vi "Place dots.vi"(6 "Right width (IMAQ height)":dbl, 8 "Left width (IMAQ height)":dbl, 9 "Right Corner":cluster{"X":sgl, "Y":sgl}[](array[cluster]), 10 "Left Corner":cluster{"X":sgl, "Y":sgl}[](array[cluster]), 11 "Image IN":T1) -> (3 "Image OUT":T1)   [LabVIEW 2018]
uses:
  <vilib>/vision/Image Controls.llb/IMAQ Image.ctl
  Dashboard globals.vi
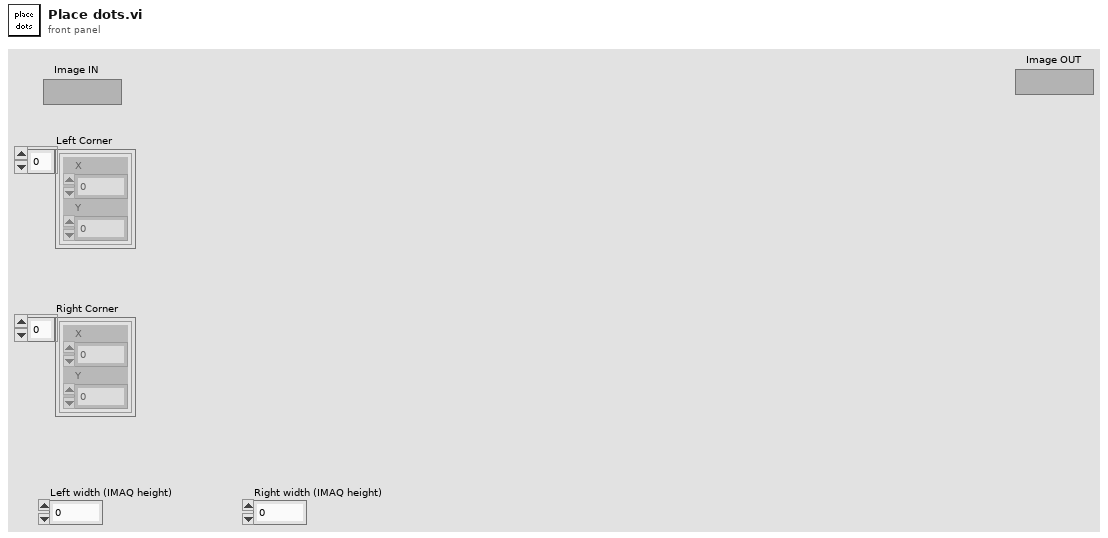
[diagram p1: front panel]
types:
  T1 = typedef "IMAQ Image.ctl" = refnum<image>
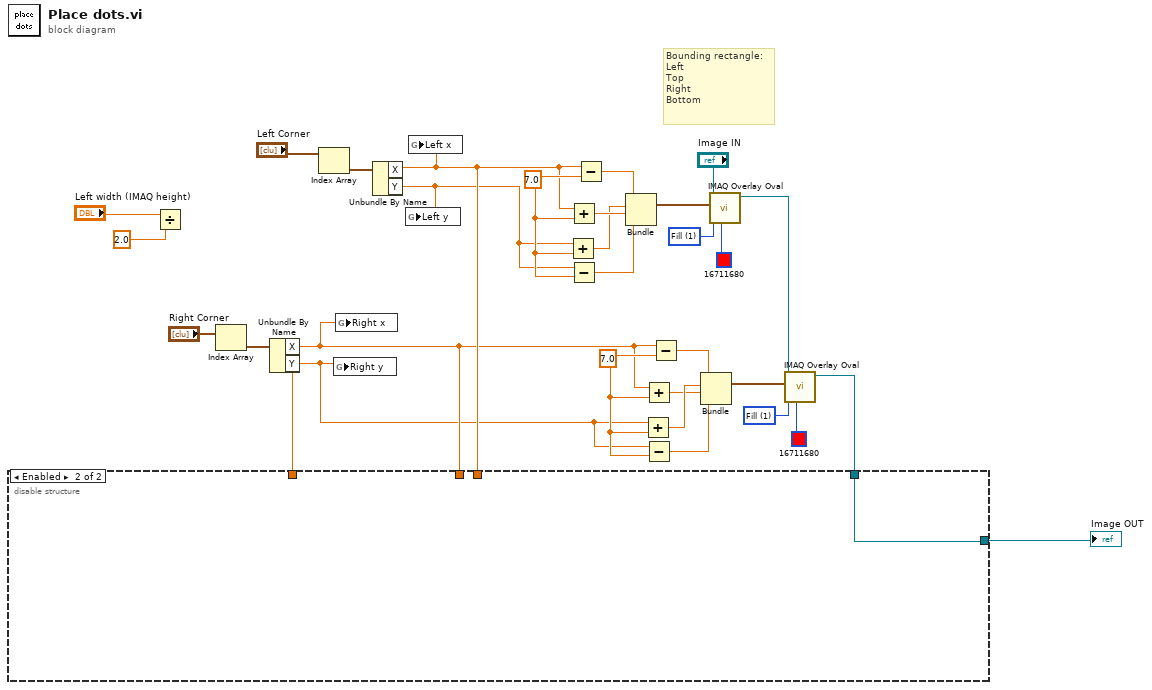
[diagram p0: block diagram]
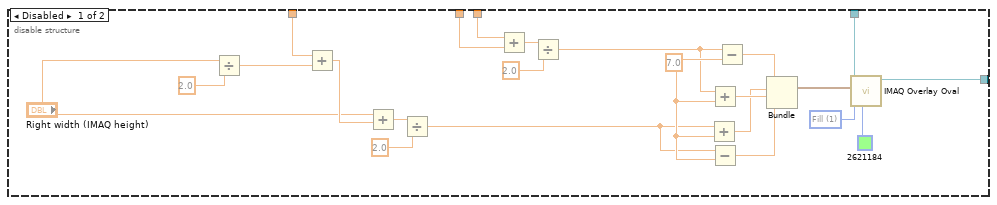
[diagram p2: hidden frame]
diagram:
  w11 = u32 1 items=["Frame", "Fill"] ("Drawing Mode (Frame)")
  w15 = sgl 7.0 ("y")
  w28 = u32 1 items=["Frame", "Fill"] ("Drawing Mode (Frame)")
  w24 = sgl 7.0 ("y")
  # "Bounding rectangle:\nLeft\nTop\nRight\nBottom"
  n1 = Divide(x="Left width (IMAQ height)", y=sgl 2.0) -> ()  [unwired: 1 out]
  n2 = Index Array(array="Right Corner") -> (element=w17:cluster{"X":sgl, "Y":sgl})  [unwired: 1 in]
  n3 = Unbundle By Name(w17) -> ("X"=w3:sgl, "Y"=w2:sgl)
  n4 = Index Array(array="Left Corner") -> (element=w20:cluster{"X":sgl, "Y":sgl})  [unwired: 1 in]
  n5 = global write "Dashboard globals.vi" "Right y"(w2) -> ()
  n6 = global write "Dashboard globals.vi" "Right x"(w3) -> ()
  n7 = Unbundle By Name(w20) -> ("X"=w4:sgl, "Y"=w1:sgl)
  n8 = global write "Dashboard globals.vi" "Left y"(w1) -> ()
  n9 = global write "Dashboard globals.vi" "Left x"(w4) -> ()
  n10 = Add(x=w1, y=w24) -> (x+y=w25:sgl)
  n11 = Add(x=w4, y=w24) -> (x+y=w26:sgl)
  n12 = Subtract(x=w1, y=w24) -> (x-y=w23:sgl)
  n13 = Subtract(x=w4, y=w24) -> (x-y=w27:sgl)
  n14 = Bundle(w27, w25, w26, w23) -> (w29:cluster{sgl, sgl, sgl, sgl})  [unwired: 1 in]
  n15 = Add(x=w2, y=w15) -> (x+y=w14:sgl)
  n16 = Add(x=w3, y=w15) -> (x+y=w13:sgl)
  n17 = Subtract(x=w2, y=w15) -> (x-y=w16:sgl)
  n18 = Subtract(x=w3, y=w15) -> (x-y=w12:sgl)
  n19 = Bundle(w12, w14, w13, w16) -> (w10:cluster{sgl, sgl, sgl, sgl})  [unwired: 1 in]
  n20 = call "IMAQ Overlay Oval"("Color"=u32 16711680 ("Side colors"), "Drawing Mode (Frame)"=w28, "Bounding Rectangle"=w29, "Image"="Image IN") -> ("Image Out"=w8:T1)  [unwired: 6 in, 1 out]
  n21 = call "IMAQ Overlay Oval"("Color"=u32 16711680 ("Side colors"), "Drawing Mode (Frame)"=w11, "Bounding Rectangle"=w10, "Image"=w8) -> ("Image Out"=w7:T1)  [unwired: 6 in, 1 out]
  n22 = disable-structure shown="Enabled" {
    disable-tunnel: w7 -> [w39 w54]
    disable-tunnel: [w38 w54] -> w6
    disable-tunnel: w4 -> [w33 _]
    disable-tunnel: w3 -> [w32 _]
    disable-tunnel: w2 -> [w31 _]
    frame Disabled {
      w52 = u32 1 items=["Frame", "Fill"] ("Drawing Mode (Frame)")
      w48 = sgl 7.0 ("y")
      n23 = Divide(x="Right width (IMAQ height)", y=sgl 2.0) -> (x/y=w36:dbl)
      n24 = Add(x=w31, y=w36) -> (x+y=w45:dbl)
      n25 = Add(x="Right width (IMAQ height)", y=w45) -> (x+y=w44:dbl)
      n26 = Divide(x=w44, y=2.0) -> (x/y=w34:dbl)
      n27 = Add(x=w33, y=w32) -> (x+y=w41:sgl)
      n28 = Divide(x=w41, y=sgl 2.0) -> (x/y=w40:sgl)
      n29 = Add(x=w34, y=w48) -> (x+y=w49:dbl)
      n30 = Add(x=w40, y=w48) -> (x+y=w50:sgl)
      n31 = Subtract(x=w34, y=w48) -> (x-y=w47:dbl)
      n32 = Subtract(x=w40, y=w48) -> (x-y=w51:sgl)
      n33 = Bundle(w51, w49, w50, w47) -> (w53:cluster{sgl, dbl, sgl, dbl})  [unwired: 1 in]
      n34 = call "IMAQ Overlay Oval"("Color"=u32 2621184 ("Side colors"), "Drawing Mode (Frame)"=w52, "Bounding Rectangle"=w53, "Image"=w39) -> ("Image Out"=w38:T1)  [unwired: 6 in, 1 out]
    }
    frame Enabled {
    }
  }
  "Image OUT" <- w6
